vi "ParameterSet.vi"(8 "error in (no error)":errorcluster, 10 "variant":variant, 11 "Module":refnum<class "ModuleAdmin.lvclass">) -> (0 "error out":errorcluster, 3 "Module out":refnum<class "ModuleAdmin.lvclass">)   [LabVIEW 2018, in "AcPwrPlugins.lvlib"]
doc: "This VI broadcasts the instrument's settings."
uses:
  AcPwrPlugins.lvlib
  <userlib>/NIST/ModuleAdminLib/ModuleAdmin/ModuleAdmin.lvclass
  AcPwrShared/clEventType.ctl
  AcPwrShared/AcPwrShared.lvlib
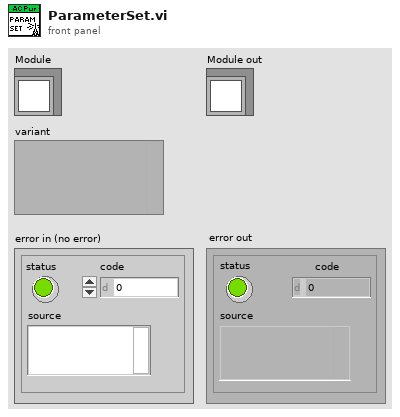
[diagram p1: front panel]
types:
  T1 = typedef "AcPwrShared.lvlib/AcPwrBroadcastEvents.ctl" = cluster{"DidInit":refnum<user-event>, "StatusUpdate":refnum<user-event>, "ErrorReport":refnum<user-event>, "DidStop":refnum<user-event>, "PathToINI":refnum<user-event>, "Measurements":refnum<user-event>, "LoadConfigFile":refnum<user-event>, "GetSettings":refnum<user-event>, "SetSettings":refnum<user-event>, "GetType&ID":refnum<user-event>, "GotSettings":refnum<user-event>, "GotSettingsLV":refnum<user-event>, "ParameterSet":refnum<user-event>}
  T2 = typedef "AcPwrShared.lvlib/clEventType.ctl" = cluster{"ModuleID":i32, "Data":variant}
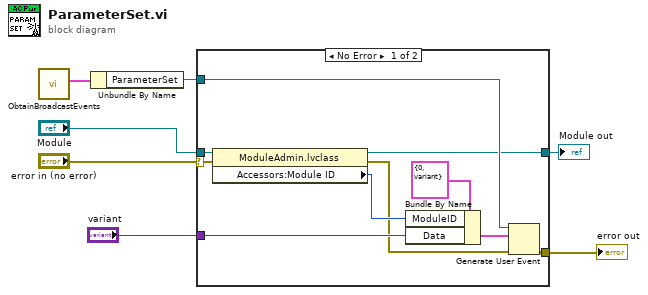
[diagram p0: block diagram]
diagram:
  n1 = call "ObtainBroadcastEvents.vi"() -> ("AcPwrEvents"=w4:T1)  [unwired: 10 in, 1 out]
  n2 = Unbundle By Name(w4) -> ("ParameterSet"=w3:refnum<user-event>)
  n3 = case shown="No Error" "error in (no error)" {
    selector: "error in (no error)" -> [w17 w19]
    tunnel: "Module" -> [w16 w18]
    tunnel: [w15 w19] -> w5
    tunnel: w3 -> [w14 _]
    tunnel: "variant" -> [w13 _]
    tunnel: [w8 w18] -> w1
    frame No Error {
      n4 = property class="ModuleAdmin.lvclass"(reference=w16, error in=w17) -> (reference out=w8:refnum<class "ModuleAdmin.lvclass">, error out=w11:errorcluster, "Accessors:Module ID"=w12:i32)
      n5 = Bundle By Name(cluster=T2 {"ModuleID"=0, "Data"=variant} ("clEventType"), "ModuleID"=w12, "Data"=w13) -> (w9:T2)
      n6 = Generate User Event(user event=w14, event data cluster=w9, error in=w11) -> (error out=w15:errorcluster)  [unwired: 1 in, 1 out]
    }
    frame Error {
    }
  }
  "error out" <- w5
  "Module out" <- w1
